vi "Test MW Delay.vi"(6 "ReadSeq W/O tw1&tw2":T3(xcontrol)=[{"Flags"=[TRUE, FALSE, TRUE, FALSE, FALSE, FALSE, FALSE, FALSE, FALSE, FALSE, FALSE, FALSE, FALSE, FALSE], "Comments"="Count1:Trigger", "Time"=1e-08, "Loop Config"={"Loop Code"=enum."Continued", "Number of Loop"=0, "End of Loop"=nan, "Loop Info"=""}}, {"Flags"=[TRUE, FALSE, FALSE, FALSE, FALSE, FALSE, FALSE, FALSE, FALSE, FALSE, FALSE, FALSE, FALSE, FALSE], "Comments"="Count1:Interval", "Time"=6e-08, "Loop Config"={"Loop Code"=enum."Continued", "Number of Loop"=0, "End of Loop"=nan, "Loop Info"=""}}, {"Flags"=[TRUE, FALSE, TRUE, FALSE, FALSE, FALSE, FALSE, FALSE, FALSE, FALSE, FALSE, FALSE, FALSE, FALSE], "Comments"="Count1:Trigger", "Time"=1e-08, "Loop Config"={"Loop Code"=enum."Continued", "Number of Loop"=0, "End of Loop"=nan, "Loop Info"=""}}, {"Flags"=[TRUE, FALSE, FALSE, FALSE, FALSE, FALSE, FALSE, FALSE, FALSE, FALSE, FALSE, FALSE, FALSE, FALSE], "Comments"="Wait", "Time"=2e-07, "Loop Config"={"Loop Code"=enum."Continued", "Number of Loop"=0, "End of Loop"=nan, "Loop Info"=""}}, {"Flags"=[TRUE, FALSE, TRUE, FALSE, FALSE, FALSE, FALSE, FALSE, FALSE, FALSE, FALSE, FALSE, FALSE, FALSE], "Comments"="Count2:Trigger", "Time"=1e-08, "Loop Config"={"Loop Code"=enum."Continued", "Number of Loop"=0, "End of Loop"=nan, "Loop Info"=""}}, {"Flags"=[TRUE, FALSE, FALSE, FALSE, FALSE, FALSE, FALSE, FALSE, FALSE, FALSE, FALSE, FALSE, FALSE, FALSE], "Comments"="Count2:Interval", "Time"=6e-08, "Loop Config"={"Loop Code"=enum."Continued", "Number of Loop"=0, "End of Loop"=nan, "Loop Info"=""}}, {"Flags"=[TRUE, FALSE, TRUE, FALSE, FALSE, FALSE, FALSE, FALSE, FALSE, FALSE, FALSE, FALSE, FALSE, FALSE], "Comments"="Count2:Trigger", "Time"=1e-08, "Loop Config"={"Loop Code"=enum."Continued", "Number of Loop"=0, "End of Loop"=nan, "Loop Info"=""}}, {"Flags"=[TRUE, FALSE, FALSE, FALSE, FALSE, FALSE, FALSE, FALSE, FALSE, FALSE, FALSE, FALSE, FALSE, FALSE], "Comments"="SupLaser", "Time"=1e-07, "Loop Config"={"Loop Code"=enum."Continued", "Number of Loop"=0, "End of Loop"=nan, "Loop Info"=""}}], 8 "error in":errorcluster, 11 "Settings":T5={"Num Pts"=350, "Freq (MHz)"=1376.0, "dBm"=6.0, "MW Delay start"=-2.5e-06, "MW Delay end"=2.5e-06, "Loop per Update"=8000, "Channel Chooser"=enum."Channel X", "AutoTrace Before Exp"=TRUE, "Update Times"=2000, "Pi"=1.3e-07} {"Pi" format="%#_6p"; "Update Times" format="%.0p"; "Loop per Update" format="%.0p"; "MW Delay end" min=-0.001 max=0.001 format="%#_6p"; "MW Delay start" format="%#_6p"; "Freq (MHz)" format="%.2f"}) -> ()   [LabVIEW 2020, in "Basic Experiment.lvlib"]
uses:
  Labview Library/Libraries/Basic Experiment/Basic Experiment.lvlib
  mw.ctl
  Labview Library/Libraries/Basic Experiment/Test MW Delay Settings.ctl
  Labview Library/Libraries/HW_LMMR_ASG8100/LMMR ASG/ASG Instructions XControl.xctl
  <vilib>/Math Plots/2D Math Plots/2D Error Bar/2D Error Bar XCtrl/2D Error Bar.xctl
  <vilib>/Math Plots/2D Math Plots/2D Error Bar/2D Error Bar Datatype/2D Error Bar Datatype.lvclass
  Labview Library/Libraries/Basic Experiment/AutoTrace Setting For Exp.ctl
  Labview Library/Libraries/HW_LMMR_ASG8100/LMMR ASG/Loop Config.ctl
  Labview Library/Libraries/HW_LMMR_ASG8100/LMMR ASG/Loop Code.ctl
  Labview Library/Libraries/Basic Experiment/Test MW Delay Result.ctl
  <vilib>/Math Plots/2D Math Plots/2D Error Bar/2D Error Bar Datatype/Public/Plot Helper (Fixed).vi
  <vilib>/express/express arith-compare/Formula/XNode/ExpressFormulaBlockNode.xnode
  Labview Library/Libraries/HW_NI_CTR/NI DAQ Counter/NI DAQ Counter.lvlib
  Labview Library/Libraries/HW_LMMR_ASG8100/LMMR ASG/ASG 8100 Module.lvlib
  Labview Library/Libraries/HW_LMMR_ASG8100/LMMR ASG/Loop XControl.xctl
  Labview Library/Libraries/HW_Rigol_DSG/Rigol Signal Generator Module/Rigol Signal Generator Module.lvlib
panel:
  in  "?":enum32{"Sequence", "PLot", "Check"}(tab)=enum."PLot"
  out "Rabi Sequence":T3(xcontrol)
  out "Total Time (min)":dbl=523.4685714285713
  in  "AutoTrace Settings":T4={"Ratio"=0.9, "Threshold"=0.009168269230769232, "Trace Times"=2, "Max Times"=100, "AutoTrace Status"=enum."Normal"}
  out "Ref WaveForm":dbl(graph)=0.00976994301994302
  in  "Stop Button":bool
  in  "Raw Seq Tab":enum32{"Channel X", "Channel Y"}(tab)
  in  "Rabi Raw Sequence X":T3(xcontrol)=[{"Flags"=[TRUE, FALSE, FALSE, FALSE, FALSE, FALSE, FALSE, FALSE, FALSE, FALSE, FALSE, FALSE, FALSE, FALSE], "Comments"="Laser", "Time"=1e-06, "Loop Config"={"Loop Code"=enum."Continued", "Number of Loop"=0, "End of Loop"=nan, "Loop Info"=""}}, {"Flags"=[FALSE, FALSE, FALSE, FALSE, FALSE, FALSE, FALSE, FALSE, FALSE, FALSE, FALSE, FALSE, FALSE, FALSE], "Comments"="tw1", "Time"=2e-06, "Loop Config"={"Loop Code"=enum."Continued", "Number of Loop"=0, "End of Loop"=nan, "Loop Info"=""}}, {"Flags"=[FALSE, TRUE, FALSE, FALSE, FALSE, FALSE, FALSE, FALSE, FALSE, FALSE, FALSE, FALSE, FALSE, FALSE], "Comments"="pi", "Time"=-1.0, "Loop Config"={"Loop Code"=enum."Continued", "Number of Loop"=0, "End of Loop"=nan, "Loop Info"=""}}, {"Flags"=[FALSE, FALSE, FALSE, FALSE, FALSE, FALSE, FALSE, FALSE, FALSE, FALSE, FALSE, FALSE, FALSE, FALSE], "Comments"="tw2", "Time"=2e-06, "Loop Config"={"Loop Code"=enum."Continued", "Number of Loop"=0, "End of Loop"=nan, "Loop Info"=""}}, {"Flags"=[TRUE, FALSE, TRUE, FALSE, FALSE, FALSE, FALSE, FALSE, FALSE, FALSE, FALSE, FALSE, FALSE, FALSE], "Comments"="ReadSeq W/O tw1&tw2", "Time"=-1.0, "Loop Config"={"Loop Code"=enum."Continued", "Number of Loop"=0, "End of Loop"=nan, "Loop Info"=""}}]
  in  "Rabi Raw Sequence Y":T3(xcontrol)=[{"Flags"=[FALSE, FALSE, FALSE, TRUE, FALSE, FALSE, FALSE, FALSE, FALSE, FALSE, FALSE, FALSE, FALSE, FALSE], "Comments"="pi", "Time"=-1.0, "Loop Config"={"Loop Code"=enum."Continued", "Number of Loop"=0, "End of Loop"=nan, "Loop Info"=""}}, {"Flags"=[FALSE, FALSE, FALSE, FALSE, FALSE, FALSE, FALSE, FALSE, FALSE, FALSE, FALSE, FALSE, FALSE, FALSE], "Comments"="tw1", "Time"=-1.0, "Loop Config"={"Loop Code"=enum."Continued", "Number of Loop"=0, "End of Loop"=nan, "Loop Info"=""}}, {"Flags"=[TRUE, FALSE, TRUE, FALSE, FALSE, FALSE, FALSE, FALSE, FALSE, FALSE, FALSE, FALSE, FALSE, FALSE], "Comments"="ReadSeq W/O tw1", "Time"=0.0, "Loop Config"={"Loop Code"=enum."Continued", "Number of Loop"=0, "End of Loop"=nan, "Loop Info"=""}}]
  out "2D Error Bar":refnum<class "2D Plot Datatype.lvclass">[](xcontrol)
  out "tau sequence":dbl[](array[numeric])=[-2.5e-06, -2.4857142857142858e-06, -2.4714285714285717e-06, -2.4571428571428573e-06, -2.4428571428571432e-06, -2.428571428571429e-06, -2.4142857142857143e-06, -2.4000000000000003e-06, -2.385714285714286e-06, -2.371428571428572e-06, -2.3571428571428574e-06, -2.342857142857143e-06, -2.328571428571429e-06, -2.3142857142857145e-06, -2.3e-06, -2.285714285714286e-06, -2.2714285714285715e-06, -2.2571428571428575e-06, -2.242857142857143e-06, -2.2285714285714286e-06, -2.2142857142857146e-06, -2.2e-06, -2.185714285714286e-06, -2.1714285714285716e-06, -2.157142857142857e-06, -2.142857142857143e-06, -2.1285714285714287e-06, -2.1142857142857143e-06, -2.1000000000000002e-06, -2.0857142857142858e-06, -2.0714285714285717e-06, -2.0571428571428573e-06, -2.042857142857143e-06, -2.028571428571429e-06, -2.0142857142857144e-06, -2.0000000000000003e-06, -1.985714285714286e-06, -1.9714285714285714e-06, -1.9571428571428574e-06, -1.942857142857143e-06, -1.9285714285714285e-06, -1.9142857142857145e-06, -1.9e-06, -1.885714285714286e-06, -1.8714285714285715e-06, -1.8571428571428573e-06, -1.842857142857143e-06, -1.8285714285714286e-06, -1.8142857142857144e-06, -1.8000000000000001e-06, -1.7857142857142857e-06, -1.7714285714285717e-06, -1.7571428571428572e-06, -1.742857142857143e-06, -1.7285714285714287e-06, -1.7142857142857143e-06, -1.7000000000000002e-06, -1.6857142857142858e-06, -1.6714285714285715e-06, -1.6571428571428573e-06, -1.6428571428571429e-06, -1.6285714285714286e-06, -1.6142857142857144e-06, -1.6e-06, -1.585714285714286e-06, -1.5714285714285714e-06, -1.5571428571428572e-06, -1.542857142857143e-06, -1.5285714285714287e-06, -1.5142857142857143e-06, -1.5e-06, -1.4857142857142858e-06, -1.4714285714285716e-06, -1.4571428571428571e-06, -1.4428571428571429e-06, -1.4285714285714286e-06, -1.4142857142857144e-06, -1.4000000000000001e-06, -1.3857142857142857e-06, -1.3714285714285715e-06, -1.3571428571428572e-06, -1.342857142857143e-06, -1.3285714285714285e-06, -1.3142857142857143e-06, -1.3e-06, -1.2857142857142858e-06, -1.2714285714285716e-06, -1.2571428571428571e-06, -1.2428571428571429e-06, -1.2285714285714286e-06, -1.2142857142857144e-06, -1.2e-06, -1.1857142857142857e-06, -1.1714285714285715e-06, -1.1571428571428572e-06, -1.1428571428571428e-06, -1.1285714285714285e-06, -1.1142857142857143e-06, -1.1e-06, -1.0857142857142858e-06, -1.0714285714285714e-06, -1.0571428571428571e-06, -1.0428571428571429e-06, -1.0285714285714286e-06, -1.0142857142857142e-06, -1e-06, -9.857142857142857e-07, -9.714285714285715e-07, -9.571428571428572e-07, -9.428571428571428e-07, -9.285714285714285e-07, -9.142857142857143e-07, -9.000000000000001e-07, -8.857142857142856e-07, -8.714285714285714e-07, -8.571428571428571e-07, -8.428571428571429e-07, -8.285714285714284e-07, -8.142857142857142e-07, -8e-07, -7.857142857142857e-07, -7.714285714285715e-07, -7.57142857142857e-07, -7.428571428571428e-07, -7.285714285714286e-07, -7.142857142857143e-07, -6.999999999999999e-07, -6.857142857142856e-07, -6.714285714285714e-07, -6.571428571428571e-07, -6.428571428571429e-07, -6.285714285714285e-07, -6.142857142857142e-07, -6e-07, -5.857142857142857e-07, -5.714285714285713e-07, -5.571428571428573e-07, -5.428571428571428e-07, -5.285714285714284e-07, -5.142857142857143e-07, -4.999999999999999e-07, -4.857142857142858e-07, -4.714285714285714e-07, -4.5714285714285694e-07, -4.428571428571429e-07, -4.2857142857142846e-07, -4.14285714285714e-07, -4e-07, -3.8571428571428553e-07, -3.714285714285715e-07, -3.5714285714285705e-07, -3.428571428571426e-07, -3.2857142857142857e-07, -3.142857142857141e-07, -3.000000000000001e-07, -2.8571428571428564e-07, -2.714285714285712e-07, -2.5714285714285716e-07, -2.428571428571427e-07, -2.2857142857142826e-07, -2.1428571428571423e-07, -1.9999999999999978e-07, -1.8571428571428575e-07, -1.714285714285713e-07, -1.5714285714285685e-07, -1.4285714285714282e-07, -1.2857142857142837e-07, -1.1428571428571434e-07, -9.999999999999989e-08, -8.571428571428544e-08, -7.142857142857141e-08, -5.714285714285696e-08, -4.285714285714293e-08, -2.857142857142848e-08, -1.4285714285714028e-08, 0.0, 1.4285714285714451e-08, 2.8571428571428903e-08, 4.285714285714293e-08, 5.714285714285738e-08, 7.142857142857141e-08, 8.571428571428586e-08, 1.0000000000000031e-07, 1.1428571428571434e-07, 1.285714285714288e-07, 1.4285714285714282e-07, 1.5714285714285727e-07, 1.7142857142857172e-07, 1.8571428571428575e-07, 2.000000000000002e-07, 2.1428571428571465e-07, 2.2857142857142868e-07, 2.4285714285714313e-07, 2.5714285714285716e-07, 2.714285714285716e-07, 2.8571428571428606e-07, 3.000000000000001e-07, 3.1428571428571454e-07, 3.2857142857142857e-07, 3.42857142857143e-07, 3.571428571428575e-07, 3.714285714285715e-07, 3.8571428571428595e-07, 4e-07, 4.1428571428571443e-07, 4.285714285714289e-07, 4.428571428571429e-07, 4.5714285714285736e-07, 4.714285714285718e-07, 4.857142857142858e-07, 5.000000000000003e-07, 5.142857142857143e-07, 5.285714285714288e-07, 5.428571428571432e-07, 5.571428571428573e-07, 5.714285714285717e-07, 5.857142857142857e-07, 6.000000000000002e-07, 6.142857142857146e-07, 6.285714285714287e-07, 6.428571428571431e-07, 6.571428571428576e-07, 6.714285714285716e-07, 6.85714285714286e-07, 7.000000000000001e-07, 7.142857142857145e-07, 7.28571428571429e-07, 7.42857142857143e-07, 7.571428571428575e-07, 7.714285714285715e-07, 7.857142857142859e-07, 8.000000000000004e-07, 8.142857142857144e-07, 8.285714285714289e-07, 8.428571428571433e-07, 8.571428571428573e-07, 8.714285714285718e-07, 8.857142857142858e-07, 9.000000000000003e-07, 9.142857142857147e-07, 9.285714285714288e-07, 9.428571428571432e-07, 9.571428571428572e-07, 9.714285714285717e-07, 9.857142857142861e-07, 1.0000000000000002e-06, 1.0142857142857146e-06, 1.0285714285714286e-06, 1.042857142857143e-06, 1.0571428571428575e-06, 1.0714285714285716e-06, 1.085714285714286e-06, 1.1000000000000005e-06, 1.1142857142857145e-06, 1.128571428571429e-06, 1.142857142857143e-06, 1.1571428571428574e-06, 1.1714285714285719e-06, 1.185714285714286e-06, 1.2000000000000004e-06, 1.2142857142857144e-06, 1.2285714285714288e-06, 1.2428571428571433e-06, 1.2571428571428573e-06, 1.2714285714285718e-06, 1.2857142857142862e-06, 1.3000000000000003e-06, 1.3142857142857147e-06, 1.3285714285714287e-06, 1.3428571428571428e-06, 1.3571428571428576e-06, 1.3714285714285717e-06, 1.3857142857142857e-06, 1.4000000000000006e-06, 1.4142857142857146e-06, 1.4285714285714286e-06, 1.4428571428571435e-06, 1.4571428571428575e-06, 1.4714285714285716e-06, 1.4857142857142864e-06, 1.5000000000000005e-06, 1.5142857142857145e-06, 1.5285714285714285e-06, 1.5428571428571434e-06, 1.5571428571428574e-06, 1.5714285714285714e-06, 1.5857142857142863e-06, 1.6000000000000004e-06, 1.6142857142857144e-06, 1.6285714285714293e-06, 1.6428571428571433e-06, 1.6571428571428573e-06, 1.6714285714285722e-06, 1.6857142857142862e-06, 1.7000000000000002e-06, 1.7142857142857143e-06, 1.7285714285714291e-06, 1.7428571428571432e-06, 1.7571428571428572e-06, 1.771428571428572e-06, 1.785714285714286e-06, 1.8000000000000001e-06, 1.814285714285715e-06, 1.828571428571429e-06, 1.842857142857143e-06, 1.857142857142858e-06, 1.871428571428572e-06, 1.885714285714286e-06, 1.9e-06, 1.914285714285715e-06, 1.928571428571429e-06, 1.942857142857143e-06, 1.957142857142858e-06, 1.971428571428572e-06, 1.985714285714286e-06, 2.0000000000000008e-06, 2.0142857142857148e-06, 2.028571428571429e-06, 2.0428571428571437e-06, 2.0571428571428577e-06, 2.0714285714285717e-06, 2.0857142857142858e-06, 2.1000000000000006e-06, 2.1142857142857147e-06, 2.1285714285714287e-06, 2.1428571428571436e-06, 2.1571428571428576e-06, 2.1714285714285716e-06, 2.1857142857142865e-06, 2.2000000000000005e-06, 2.2142857142857146e-06, 2.2285714285714286e-06, 2.2428571428571435e-06, 2.2571428571428575e-06, 2.2714285714285715e-06, 2.2857142857142864e-06, 2.3000000000000004e-06, 2.3142857142857145e-06, 2.3285714285714293e-06, 2.3428571428571434e-06, 2.3571428571428574e-06, 2.3714285714285723e-06, 2.3857142857142863e-06, 2.4000000000000003e-06, 2.4142857142857143e-06, 2.4285714285714292e-06, 2.4428571428571432e-06, 2.4571428571428573e-06, 2.471428571428572e-06, 2.485714285714286e-06, 2.5e-06]
  out "Signal Sum":dbl[](array[numeric])=[-0.0, -0.0, -0.0, -0.0, -0.0, -0.0, -0.0, -0.0, -0.0, -0.0, -0.0, -0.0, -0.0, -0.0, -0.0, -0.0, -0.0, -0.0, -0.0, -0.0, -0.0, -0.0, -0.0, -0.0, -0.0, -0.0, -0.0, -0.0, -0.0, -0.0, -0.0, -0.0, -0.0, -0.0, -0.0, -0.0, -0.0, -0.0, -0.0, -0.0, -0.0, -0.0, -0.0, -0.0, -0.0, -0.0, -0.0, -0.0, -0.0, -0.0, -0.0, -0.0, -0.0, -0.0, -0.0, -0.0, -0.0, -0.0, -0.0, -0.0, -0.0, -0.0, -0.0, -0.0, -0.0, -0.0, -0.0, -0.0, -0.0, -0.0, -0.0, -0.0, -0.0, -0.0, -0.0, -0.0, -0.0, -0.0, -0.0, -0.0, -0.0, -0.0, -0.0, -0.0, -0.0, -0.0, -0.0, -0.0, -0.0, -0.0, -0.0, -0.0, -0.0, -0.0, -0.0, -0.0, -0.0, -0.0, -0.0, -0.0, -0.0, -0.0, -0.0, -0.0, -0.0, -0.0, -0.0, -0.0, -0.0, -0.0, -0.0, -0.0, -0.0, -0.0, -0.0, -0.0, -0.0, -0.0, -0.0, -0.0, -0.0, -0.0, -0.0, -0.0, -0.0, -0.0, -0.0, -0.0, -0.0, -0.0, -0.0, -0.0, -0.0, -0.0, -0.0, -0.0, -0.0, -0.0, -0.0, -0.0, -0.0, -0.0, -0.0, -0.0, -0.0, -0.0, -0.0, -0.0, -0.0, -0.0, -0.0, -0.0, -0.0, -0.0, -0.0, -0.0, -0.0, -0.0, -0.0, -0.0, -0.0, -0.0, -0.0, -0.0, -0.0, -0.0, -0.0, -0.0, -0.0, -0.0, -0.0, -0.0, -0.0, -0.0, -0.0, 0.0, 0.0, 0.0, 0.0, 0.0, 0.0, 0.0, 0.0, 0.0, 0.0, 0.0, 0.0, 0.0, 0.0, 0.0, 0.0, 0.0, 0.0, 0.0, 0.0, 0.0, 0.0, 0.0, 0.0, 0.0, 0.0, 0.0, 0.0, 0.0, 0.0, 0.0, 0.0, 0.0, 0.0, 0.0, 0.0, 0.0, 0.0, 0.0, 0.0, 0.0, 0.0, 0.0, 0.0, 0.0, 0.0, 0.0, 0.0, 0.0, 0.0, 0.0, 0.0, 0.0, 0.0, 0.0, 0.0, 0.0, 0.0, 0.0, 0.0, 0.0, 0.0, 0.0, 0.0, 0.0, 0.0, 0.0, 0.0, 0.0, 0.0, 0.0, 0.0, 0.0, 0.0, 0.0, 0.0, 0.0, 0.0, 0.0, 0.0, 0.0, 0.0, 0.0, 0.0, 0.0, 0.0, 0.0, 0.0, 0.0, 0.0, 0.0, 0.0, 0.0, 0.0, 0.0, 0.0, 0.0, 0.0, 0.0, 0.0, 0.0, 0.0, 0.0, 0.0, 0.0, 0.0, 0.0, 0.0, 0.0, 0.0, 0.0, 0.0, 0.0, 0.0, 0.0, 0.0, 0.0, 0.0, 0.0, 0.0, 0.0, 0.0, 0.0, 0.0, 0.0, 0.0, 0.0, 0.0, 0.0, 0.0, 0.0, 0.0, 0.0, 0.0, 0.0, 0.0, 0.0, 0.0, 0.0, 0.0, 0.0, 0.0, 0.0, 0.0, 0.0, 0.0, 0.0, 0.0, 0.0, 0.0, 0.0, 0.0, 0.0, 0.0, 0.0, 0.0, 0.0, 0.0, 0.0, 0.0, 0.0, 0.0, 0.0, 0.0, 0.0, 0.0, 0.0, 0.0, 0.0, 0.0, 0.0, 0.0, 0.0, 0.0, 0.0, 0.0]
  out "error out":errorcluster
  out "Ref Sum":dbl[](array[numeric])=[-0.0, -0.0, -0.0, -0.0, -0.0, -0.0, -0.0, -0.0, -0.0, -0.0, -0.0, -0.0, -0.0, -0.0, -0.0, -0.0, -0.0, -0.0, -0.0, -0.0, -0.0, -0.0, -0.0, -0.0, -0.0, -0.0, -0.0, -0.0, -0.0, -0.0, -0.0, -0.0, -0.0, -0.0, -0.0, -0.0, -0.0, -0.0, -0.0, -0.0, -0.0, -0.0, -0.0, -0.0, -0.0, -0.0, -0.0, -0.0, -0.0, -0.0, -0.0, -0.0, -0.0, -0.0, -0.0, -0.0, -0.0, -0.0, -0.0, -0.0, -0.0, -0.0, -0.0, -0.0, -0.0, -0.0, -0.0, -0.0, -0.0, -0.0, -0.0, -0.0, -0.0, -0.0, -0.0, -0.0, -0.0, -0.0, -0.0, -0.0, -0.0, -0.0, -0.0, -0.0, -0.0, -0.0, -0.0, -0.0, -0.0, -0.0, -0.0, -0.0, -0.0, -0.0, -0.0, -0.0, -0.0, -0.0, -0.0, -0.0, -0.0, -0.0, -0.0, -0.0, -0.0, -0.0, -0.0, -0.0, -0.0, -0.0, -0.0, -0.0, -0.0, -0.0, -0.0, -0.0, -0.0, -0.0, -0.0, -0.0, -0.0, -0.0, -0.0, -0.0, -0.0, -0.0, -0.0, -0.0, -0.0, -0.0, -0.0, -0.0, -0.0, -0.0, -0.0, -0.0, -0.0, -0.0, -0.0, -0.0, -0.0, -0.0, -0.0, -0.0, -0.0, -0.0, -0.0, -0.0, -0.0, -0.0, -0.0, -0.0, -0.0, -0.0, -0.0, -0.0, -0.0, -0.0, -0.0, -0.0, -0.0, -0.0, -0.0, -0.0, -0.0, -0.0, -0.0, -0.0, -0.0, -0.0, -0.0, -0.0, -0.0, -0.0, -0.0, 0.0, 0.0, 0.0, 0.0, 0.0, 0.0, 0.0, 0.0, 0.0, 0.0, 0.0, 0.0, 0.0, 0.0, 0.0, 0.0, 0.0, 0.0, 0.0, 0.0, 0.0, 0.0, 0.0, 0.0, 0.0, 0.0, 0.0, 0.0, 0.0, 0.0, 0.0, 0.0, 0.0, 0.0, 0.0, 0.0, 0.0, 0.0, 0.0, 0.0, 0.0, 0.0, 0.0, 0.0, 0.0, 0.0, 0.0, 0.0, 0.0, 0.0, 0.0, 0.0, 0.0, 0.0, 0.0, 0.0, 0.0, 0.0, 0.0, 0.0, 0.0, 0.0, 0.0, 0.0, 0.0, 0.0, 0.0, 0.0, 0.0, 0.0, 0.0, 0.0, 0.0, 0.0, 0.0, 0.0, 0.0, 0.0, 0.0, 0.0, 0.0, 0.0, 0.0, 0.0, 0.0, 0.0, 0.0, 0.0, 0.0, 0.0, 0.0, 0.0, 0.0, 0.0, 0.0, 0.0, 0.0, 0.0, 0.0, 0.0, 0.0, 0.0, 0.0, 0.0, 0.0, 0.0, 0.0, 0.0, 0.0, 0.0, 0.0, 0.0, 0.0, 0.0, 0.0, 0.0, 0.0, 0.0, 0.0, 0.0, 0.0, 0.0, 0.0, 0.0, 0.0, 0.0, 0.0, 0.0, 0.0, 0.0, 0.0, 0.0, 0.0, 0.0, 0.0, 0.0, 0.0, 0.0, 0.0, 0.0, 0.0, 0.0, 0.0, 0.0, 0.0, 0.0, 0.0, 0.0, 0.0, 0.0, 0.0, 0.0, 0.0, 0.0, 0.0, 0.0, 0.0, 0.0, 0.0, 0.0, 0.0, 0.0, 0.0, 0.0, 0.0, 0.0, 0.0, 0.0, 0.0, 0.0, 0.0, 0.0, 0.0, 0.0, 0.0, 0.0]
  in  "MW":T6={"mw_source"=enum."rigol", "MW Source IP Address"="169.254.101.2", "Remote Port"=5025, "Frequency(MHz)"=1376.0, "Power(dBm)"=6.0}
  # "Test MW Delay Settings"
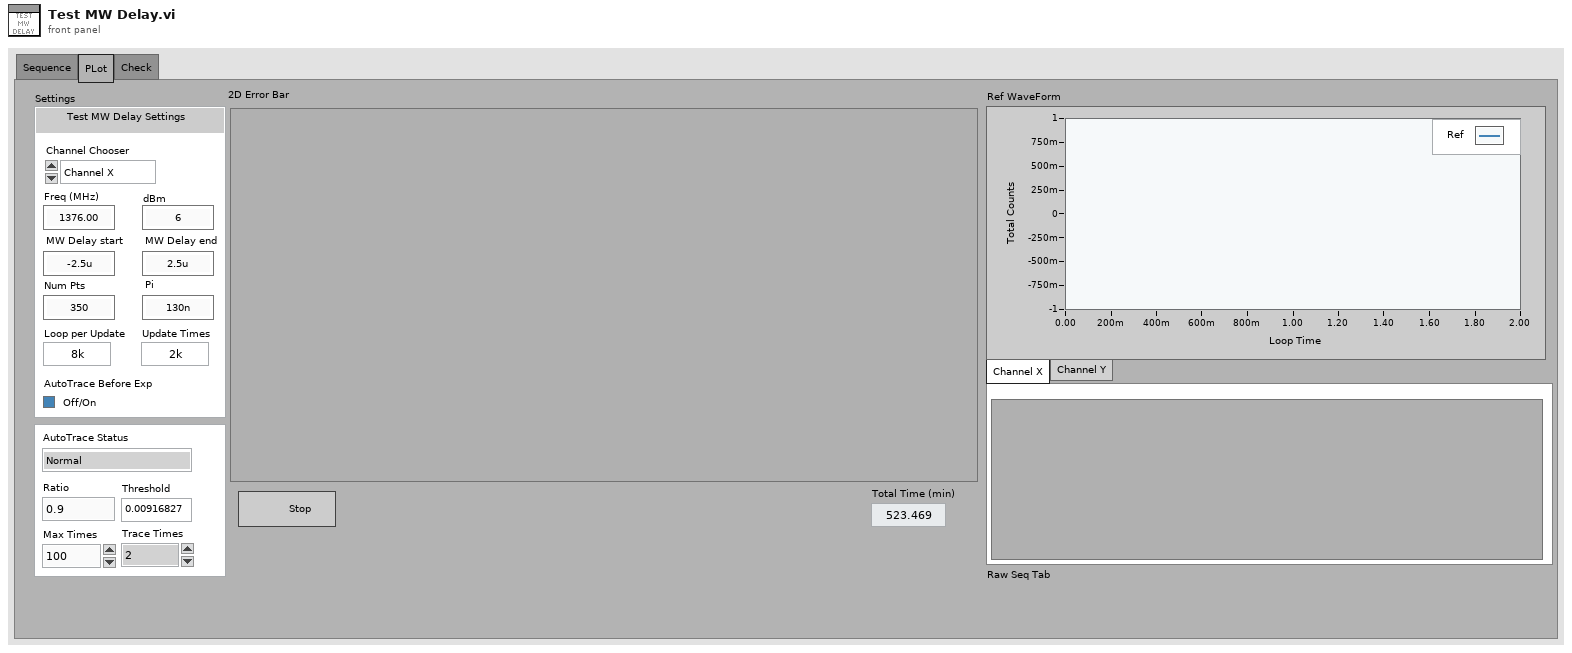
[diagram p1: front panel]
types:
  T1 = typedef "Loop XControl.xctl/Loop Config.ctl" = cluster{"Loop Code":T2, "Number of Loop":i32, "End of Loop":dbl, "Loop Info":string}
  T2 = typedef "Loop XControl.xctl/Loop Code.ctl" = enum16{"Continued", "Loop", "End Loop"}
  T3 = cluster{"Flags":bool[], "Comments":string, "Time":dbl, "Loop Config":T1}[]
  T4 = typedef "Basic Experiment.lvlib/AutoTrace Setting For Exp.ctl" = cluster{"Ratio":dbl, "Threshold":dbl, "Trace Times":i32, "Max Times":i32, "AutoTrace Status":enum16{"Normal", "AutoTrace  Last Loop", "Unintialized"}}
  T5 = typedef "Basic Experiment.lvlib/Test MW Delay Settings.ctl" = cluster{"Num Pts":i32, "Freq (MHz)":dbl, "dBm":dbl, "MW Delay start":dbl, "MW Delay end":dbl, "Loop per Update":u32, "Channel Chooser":enum16{"Channel X", "Channel Y"}, "AutoTrace Before Exp":bool, "Update Times":u32, "Pi":dbl}
  T6 = typedef "mw.ctl" = cluster{"mw_source":enum16{"rigol", "stanford", "apsin", "hittle"}, "MW Source IP Address":string, "Remote Port":u16, "Frequency(MHz)":dbl, "Power(dBm)":dbl}
  T7 = enum16{"Normal", "AutoTrace  Last Loop", "Unintialized"}
  T8 = enum16{"open", "open or create", "create or replace", "create", "open (read-only)"}
  T9 = typedef "Basic Experiment.lvlib/Test MW Delay Result.ctl" = cluster{"Pro":dbl[], "Raw Tdms Path":path, "Raw Image Path":path, "ErrorBar":dbl[]}
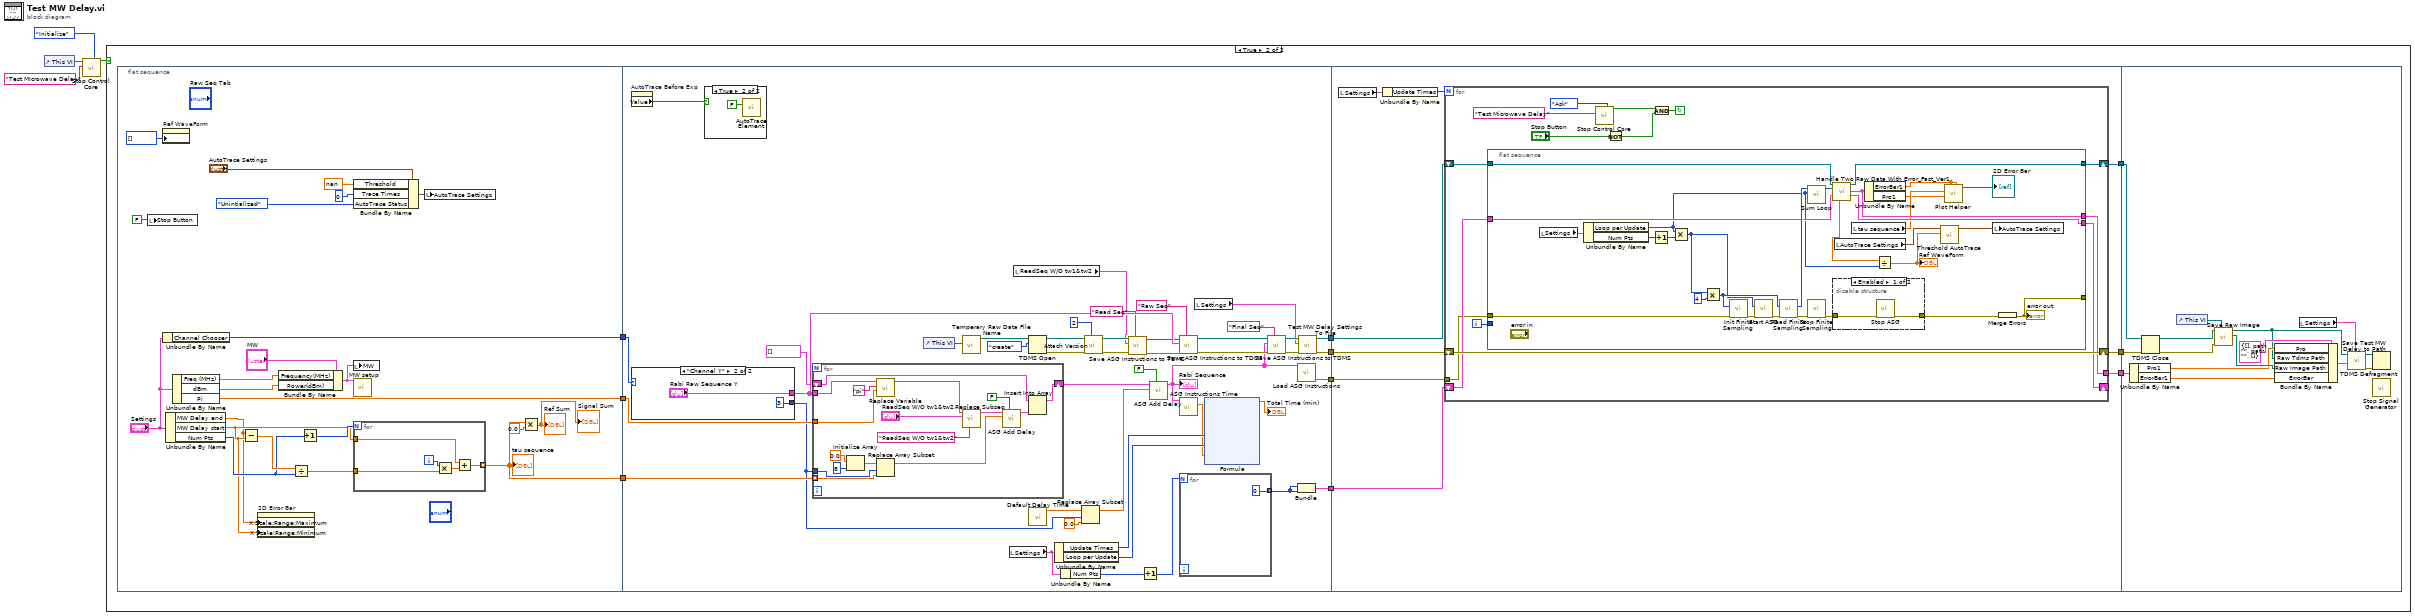
[diagram p0: block diagram]
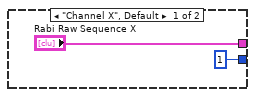
[diagram p3: hidden frame]
diagram:
  n1 = control-ref of="This VI"() -> (w3:refnum<vi>)
  n2 = call "Stop Control Core.vi"("Mode"=enum16{"Ask", "Initialize"}."Initialize", "Program Name"="Test MIcrowave Delay", "VI Ref"=w3) -> ("Continue Sign(Continue:True)"=w1:bool)  [unwired: 8 in]
  n3 = case shown="True" w1 {
    frame False {
    }
    frame True {
      n4 = flat-sequence {
        tunnel: [w26] -> w14
        tunnel: [w24] -> w13
        tunnel: [w18] -> w7
        tunnel: w14 -> [w86]
        tunnel: [w75] -> w12
        tunnel: [w74] -> w11
        tunnel: w13 -> [w73]
        tunnel: w7 -> [w65]
        tunnel: [w51] -> w6
        tunnel: [w50] -> w5
        tunnel: w12 -> [w129]
        tunnel: w11 -> [w130]
        tunnel: [w128] -> w10
        tunnel: [w127] -> w9
        tunnel: [w126] -> w8
        tunnel: w6 -> [w125]
        tunnel: w5 -> [w124]
        tunnel: w8 -> [w184]
        tunnel: w9 -> [w187]
        tunnel: w10 -> [w188]
        frame #0 {
          n5 = local write "Stop Button"(FALSE) -> ()
          n6 = property on="Ref WaveForm" class="WFChart (strict)"("History Data"=u32[] []) -> ()  [unwired: 2 in, 2 out]
          n7 = Unbundle By Name("Settings") -> ("Channel Chooser"=w24:enum16{"Channel X", "Channel Y"})
          n8 = Unbundle By Name("Settings") -> ("MW Delay end"=w15:dbl, "MW Delay start"=w16:dbl, "Num Pts"=w34:i32)
          n9 = Unbundle By Name("Settings") -> ("Freq (MHz)"=w31:dbl, "dBm"=w32:dbl, "Pi"=w18:dbl)
          n10 = Subtract(x=w15, y=w16) -> (x-y=w35:dbl)
          n11 = property on="2D Error Bar" class="2D Error Bar (strict)"("X Scale:Range:Maximum"=w15, "X Scale:Range:Minimum"=w16) -> ()  [unwired: 2 in, 2 out]
          n12 = Bundle By Name(cluster="MW", "Frequency(MHz)"=w31, "Power(dBm)"=w32) -> (w30:T6)
          n13 = Divide(x=w35, y=w34) -> (x/y=w37:dbl)
          n14 = Increment(x=w34) -> (x+1=w36:i32)
          n15 = Bundle By Name(cluster="AutoTrace Settings", "Threshold"=nan, "Trace Times"=0, "AutoTrace Status"=T7."Unintialized" ("Value")) -> (w19:T4)
          n16 = local write "MW"(w30) -> ()
          n17 = call "MW setup.vi"("mw"=w30) -> ()  [unwired: 11 in]
          n18 = for {
            N: w36 -> [_]
            tunnel: w16 -> [w41]
            tunnel: w37 -> [w42]
            tunnel: [w38] -> w26 mode=indexing
            i -> [w39]
            n19 = Multiply(x=w39, y=w42) -> (x*y=w40:dbl)
            n20 = Add(x=w41, y=w40) -> (x+y=w38:dbl)
          }
          "tau sequence" <- w26
          n21 = local write "AutoTrace Settings"(w19) -> ()
          n22 = Multiply(x=w26, y=0.0) -> (x*y=→"Signal Sum" →"Ref Sum":dbl[])
        }
        frame #1 {
          n23 = property on="AutoTrace Before Exp" class="Bool (strict)"() -> ("Value"=w69:bool)  [unwired: 2 in, 2 out]
          n24 = case shown="\"Channel Y\"" w73 {
            tunnel: ["Rabi Raw Sequence X" "Rabi Raw Sequence Y"] -> w78
            tunnel: [1 ("dimension size") 3 ("index")] -> w62
            frame "Channel X", Default {
            }
            frame "Channel Y" {
            }
          }
          n25 = case shown="True" w69 {
            frame False {
            }
            frame True {
              n26 = call "AutoTrace Element.vi"("Need Correct Count?(T)"=FALSE) -> ()  [unwired: 9 in, 2 out]
            }
          }
          n27 = for {
            tunnel: w86 -> [w106] mode=indexing
            tunnel: w78 -> [w120]
            shift-right: [w118] -> w64
            shift-left: T3 [] ("Rabi Raw Sequence") -> [w119]
            tunnel: w65 -> [w114]
            tunnel: w62 -> [w105]
            n28 = Initialize Array(0.0 ("element"), 8 ("dimension size")) -> (w109:dbl[])
            n29 = call "Replace Variable.vi"("Variable value"=w114, "Variable Name"="pi", "Seq"=w120) -> ("Result seq"=w113:T3)  [unwired: 8 in]
            n30 = Replace Array Subset(array=w109, new element=w106, index=w105) -> (w104:dbl[])
            n31 = call "Replace Subseq.vi"("SubSeq Name"="ReadSeq W/O tw1&tw2", "SubSeq"="ReadSeq W/O tw1&tw2", "Seq"=w113) -> ("Result Seq"=w112:T3)  [unwired: 8 in]
            n32 = call "ASG Add Delay.vi"("Round Time (to 1ns Precision)(TRUE)"=FALSE, "Channel delays(s)"=w104, "Input Sequence"=w112) -> ("Output Sequence"=w111:T3)  [unwired: 7 in, 1 out]
            n33 = Insert Into Array(array=w119, new element=w111) -> (w118:T3)  [unwired: 1 in]
          }
          n34 = control-ref of="This VI"() -> (w83:refnum<vi>)
          n35 = call "Temperary Raw Data File Name.vi"("VI ref"=w83) -> ("Raw data Path"=w79:path)  [unwired: 10 in]
          n36 = local read "Settings"() -> (w54:T5)
          n37 = local read "ReadSeq W/O tw1&tw2"() -> (w43:T3)
          n38 = TDMS Open(10:T8."create" ("operation (0:open)"), 11:w79) -> (0:w72:errorcluster, 3:w71:refnum<k34>)  [unwired: 5 in]
          n39 = call "Default Delay Time.vi"() -> ("Delay Time"=w63:dbl[])  [unwired: 10 in, 1 out]
          n40 = Unbundle By Name(w54) -> ("Update Times"=w58:u32, "Loop per Update"=w57:u32)
          n41 = Unbundle By Name(w54) -> ("Num Pts"=w55:i32)
          n42 = Replace Array Subset(array=w63, new element=0.0 ("new element/subarray"), index=w62) -> (w60:dbl[])
          n43 = call "Attach Version.vi"("Version"=u32 2, "error in (no error)"=w72, "Refnum in"=w71) -> ("error out"=w48:errorcluster, "Refnum out"=w46:refnum<k34>)  [unwired: 5 in, 2 out]
          n44 = call "Save ASG Instructions to TDMS.vi"("Name"="Read Seq", "error in (no error)"=w48, "ASG Instructions"=w43, "tdms file"=w46) -> ("error out"=w47:errorcluster, "tdms file out"=w45:refnum<k34>)  [unwired: 6 in]
          n45 = Increment(x=w55) -> (x+1=w53:i32)
          n46 = call "ASG Add Delay.vi"("Round Time (to 1ns Precision)(TRUE)"=FALSE, "Channel delays(s)"=w60, "Input Sequence"=w64) -> ("Output Sequence"=w67:T3)  [unwired: 7 in, 1 out]
          "Rabi Sequence" <- w67
          n47 = call "Save ASG Instructions to TDMS.vi"("Name"="Raw Seq", "error in (no error)"=w47, "ASG Instructions"=w78, "tdms file"=w45) -> ("error out"=w80:errorcluster, "tdms file out"=w81:refnum<k34>)  [unwired: 6 in]
          n48 = call "ASG Instructions Time.vi"("ASG Instr. A"=w67) -> ("Total Time (s)"=w56:ext)  [unwired: 10 in]
          n49 = for {
            N: w53 -> [_]
            tunnel: [0] -> w52 mode=indexing
          }
          n50 = local read "Settings"() -> (w49:T5)
          n51 = xnode "Formula"("Update Time"=w58, "Loop per Update"=w57, "Seq Time"=w56) -> ("Result"=→"Total Time (min)":ext)  [unwired: 1 in, 1 out]
          n52 = call "Save ASG Instructions to TDMS.vi"("Name"="Final Seq", "error in (no error)"=w80, "ASG Instructions"=w67, "tdms file"=w81) -> ("error out"=w76:errorcluster, "tdms file out"=w77:refnum<k34>)  [unwired: 6 in]
          n53 = call "Load ASG Instructions.vi"("ASG Instructions"=w67) -> ("error out"=w51:errorcluster)  [unwired: 10 in]
          n54 = Bundle(w52, w52) -> (w50:cluster{i32[], i32[]})  [unwired: 1 in]
          n55 = call "Test MW Delay Settings To File.vi"("error in (no error)"=w76, "Settings"=w49, "tdms file"=w77) -> ("error out"=w74:errorcluster, "tdms file out"=w75:refnum<k34>)  [unwired: 7 in]
        }
        frame #2 {
          n56 = local read "Settings"() -> (w123:T5)
          n57 = Unbundle By Name(w123) -> ("Update Times"=w122:u32)
          n58 = for {
            N: w122 -> [_]
            shift-right: [w139] -> w127
            shift-left: w129 -> [w140]
            shift-right: [w143] -> w128
            shift-left: w130 -> [w143]
            shift-right: [w142] -> _
            shift-left: w124 -> [w141]
            tunnel: [w136] -> w126
            tunnel: w125 -> [w131]
            i -> [w144]
            stop <- w132 continue-if-true
            n59 = flat-sequence {
              tunnel: [w173] -> w142
              tunnel: [w172] -> w136
              tunnel: w131 -> [w167]
              tunnel: [w159] -> _
              tunnel: w141 -> [w157]
              tunnel: w140 -> [w156]
              tunnel: [w155] -> w139
              tunnel: w144 -> [_]
              frame #0 {
                n60 = local read "Settings"() -> (w171:T5)
                n61 = Unbundle By Name(w171) -> ("Loop per Update"=w149:u32, "Num Pts"=w162:i32)
                n62 = Increment(x=w162) -> (x+1=w160:i32)
                n63 = Multiply(x=w149, y=w160) -> (x*y=w161:u32)
                n64 = Multiply(x=w161, y=4) -> (x*y=w169:u32)
                n65 = call "Init Finite Sampling.vi"("error in"=w167, "Num of Sample"=w169) -> ("error out"=w164:errorcluster)  [unwired: 9 in]
                n66 = call "Start ASG.vi"("error in (no error)"=w164, "Loop Number"=w161) -> ("error out"=w163:errorcluster)  [unwired: 8 in, 1 out]
                n67 = call "Read Finite Sampling.vi"("error in"=w163, "Samples to Read"=w169) -> ("error out"=w170:errorcluster, "Sample Array"=w158:u32[])  [unwired: 7 in, 1 out]
                n68 = call "Sum Loop.vi"("Loop per Update"=w149, "Raw Data Array"=w158) -> ("Data after sum"=w151:u32[])  [unwired: 9 in]
                n69 = call "Stop Finite Sampling.vi"("error in"=w170) -> ("error out"=w166:errorcluster)  [unwired: 10 in]
                n70 = call "Handle Two Raw Data With Error_Fast_Ver1.vi"("Refnum in"=w156, "TwoTypeRawData"=w151, "Storage"=w157) -> ("tdms file out"=w155:refnum<k34>, "Result"=w172:cluster{"Pro1":dbl[], "ErrorBar1":dbl[]}, "New Storage"=w173:cluster{"Sig1":u32[], "Ref1":u32[]}, "mean"=w148:dbl)  [unwired: 8 in, 1 out]
                n71 = disable-structure shown="Enabled" {
                  disable-tunnel: w166 -> [w175 w176]
                  disable-tunnel: [w174 w176] -> w165
                  frame Enabled {
                    n72 = call "Stop ASG.vi"("error in (no error)"=w175) -> ("error out"=w174:errorcluster)  [unwired: 9 in, 1 out]
                  }
                  frame Disabled {
                  }
                }
                n73 = local read "AutoTrace Settings"() -> (w146:T4)
                n74 = local read "tau sequence"() -> (w154:dbl[])
                n75 = Unbundle By Name(w172) -> ("ErrorBar1"=w152:dbl[], "Pro1"=w150:dbl[])
                n76 = Divide(x=w148, y=w149) -> (x/y=w147:dbl)
                "Ref WaveForm" <- w147
                n77 = call "Threshold AutoTrace.vi"("Count"=w147, "AutoTrace Settings In"=w146) -> ("AutoTrace Settings Out"=w145:T4)  [unwired: 9 in]
                n78 = call-poly <vilib>:"Plot Helper.vi"("error b vector"=w152, "error a vector"=w152, "y vector"=w150, "x vector"=w154) -> ("2D Plot Class Obj Array out"=→"2D Error Bar":refnum<class "2D Plot Datatype.lvclass">[])  [unwired: 2 in, 5 out]
                n79 = local write "AutoTrace Settings"(w145) -> ()
                n80 = Merge Errors(w165) -> (w159:errorcluster)
                "error out" <- w159
              }
            }
            n81 = call "Stop Control Core.vi"("Mode"=enum16{"Ask", "Initialize"}."Ask", "Program Name"="Test Microwave Delay") -> ("Continue Sign(Continue:True)"=w133:bool)  [unwired: 9 in]
            n82 = Not(x="Stop Button") -> (.not. x?=w134:bool)
            n83 = And(x=w133, y=w134) -> (x .and. y?=w132:bool)
          }
        }
        frame #3 {
          n84 = Unbundle By Name(w184) -> ("Pro1"=w183:dbl[], "ErrorBar1"=w182:dbl[])
          n85 = TDMS Close(8:w188, 11:w187) -> (0:w190:errorcluster, 3:w189:path)
          n86 = control-ref of="This VI"() -> (w191:refnum<vi>)
          n87 = call "Save Raw Image.vi"("reference"=w191, "error in"=w190, "Raw TDMS Path"=w189) -> ("Image Path"=w185:path, "Raw TDMS Path Out"=w181:path)  [unwired: 6 in, 1 out]
          n88 = Bundle By Name(cluster=T9 {"Pro"=[], "Raw Tdms Path"=path "", "Raw Image Path"=path "", "ErrorBar"=[]} ("Rabi Results"), "Pro"=w183, "Raw Tdms Path"=w181, "Raw Image Path"=w185, "ErrorBar"=w182) -> (w180:T9)
          n89 = local read "Settings"() -> (w179:T5)
          n90 = call "Save Test MW Delay to Path.vi"("Settings"=w179, "Rabi Results"=w180, "file path"=w181) -> ("error out"=w177:errorcluster, "tdms path out"=w178:path)  [unwired: 5 in, 2 out]
          n91 = TDMS Defragment(4:w177, 7:w178) -> ()  [unwired: 1 out]
          n92 = call "Stop Signal Generator.vi"() -> ()  [unwired: 10 in, 2 out]
        }
      }
    }
  }
